vi "State Convert for Save.vi"(6 "Control Ref Queue":T1, 8 "error in (no error)":errorcluster, 11 "2D Plot.lvclass":refnum<class "2D Plot.lvclass">) -> (0 "error out":errorcluster, 1 "Plot Legend Color":u32(colorbox), 2 "Main Frame Color":u32(colorbox), 3 "2D Plot.lvclass out":refnum<class "2D Plot.lvclass">)   [LabVIEW 2017, in "2D Plot.lvclass"]
uses:
  <vilib>/Math Plots/2D Math Plots/2D Plot/2D Plot/2D Plot.lvclass
  <vilib>/Math Plots/2D Math Plots/2D Plot/Action String/2DMathPlot Ctrl Act Queue.ctl
  <vilib>/Math Plots/2D Math Plots/2D Plot/Action String/2DMathPlot Ctrl Act Cluster.ctl
  <vilib>/Math Plots/2D Math Plots/2D Plot/Action String/2DMathPlot State Class.ctl
  <vilib>/Math Plots/2D Math Plots/2D Plot/2D Plot/2D Plot.lvclass/2D Plot.ctl
  <vilib>/Math Plots/Plot Private Lib/NI_Math Plot Private Lib.lvlib
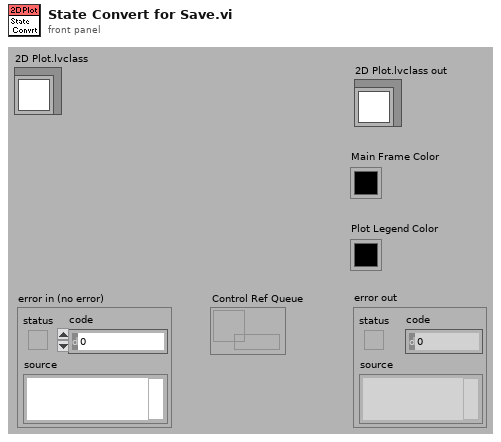
[diagram p1: front panel]
types:
  T1 = typedef "2DMathPlot Ctrl Act Queue.ctl" = refnum<queue>
  T2 = typedef "2DMathPlot Ctrl Act Cluster.ctl" = cluster{"Plot Area Ref":refnum<vi>, "Z Axis Ref":refnum<vi>, "Legend Ref":refnum<vi>, "XControl Ref":refnum<vi>, "Facade Ref":refnum<vi>, "Display State Change Class":T3}
  T3 = typedef "2DMathPlot State Class.ctl" = enum16{"Update All (Undo)", "Update General", "Update Appearance", "Update Format", "Update Scale", "Update Marker", "Update Cursor", "None"}
  T4 = typedef "LVRectTypeDef.ctl" = cluster{"Left":i16, "Top":i16, "Right":i16, "Bottom":i16}
  T5 = typedef "LVAnnotationListTypeDef.ctl" = cluster{"Name":string, "Color":u32, "Style":u8, "Point Style":u8, "Name Visible":bool, "Allow Drag":bool, "Annotation Mode":u32, "Plot":i32, "Index":i32, "Position":cluster{"X":dbl, "Y":dbl}, "X Scale":u32, "Y Scale":u32, "Show Arrow":bool, "Lock Name":bool, "Plot Area":i32, "Label Offset":cluster{"X":dbl, "Y":dbl}}[]
  T6 = typedef "LVCursorListTypeDef.ctl" = cluster{"Name":string, "Color":u32, "Style":u8, "Point Style":u8, "Name Visible":bool, "Allow Drag":bool, "Cursor Mode":u32, "Plot":i32, "Index":i32, "Position":cluster{"X":dbl, "Y":dbl}, "X Scale":u32, "Y Scale":u32, "Watch Plots":i32[], "Watch All Plots":bool, "Plot Area":i32, "Label Offset":cluster{"X":dbl, "Y":dbl}}[]
  T7 = cluster{"Cursor Selection Color":u32, "Line Style":u8, "Line Width":u8, "Visible":bool}
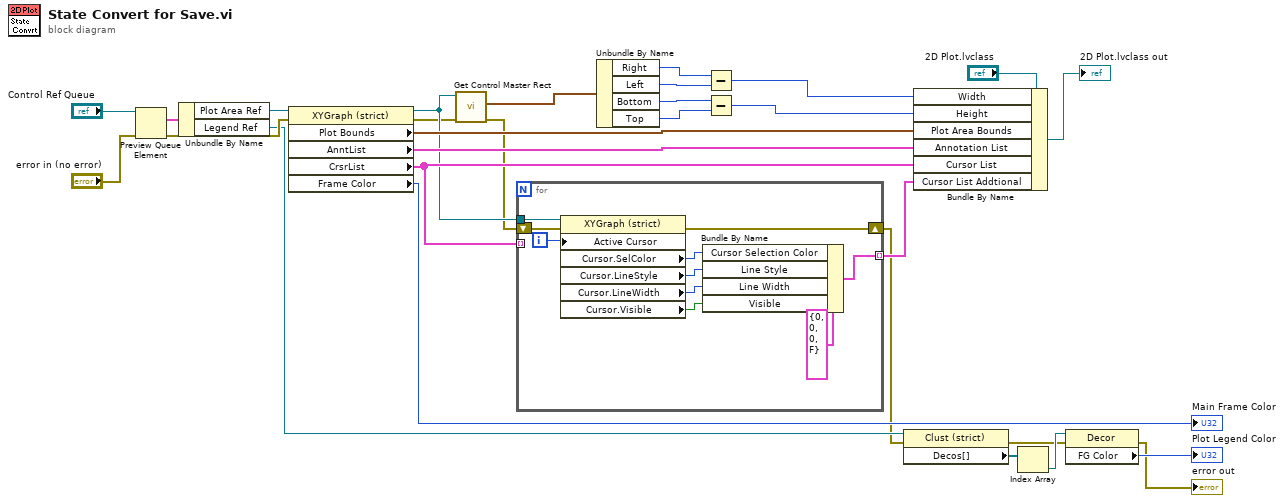
[diagram p0: block diagram]
diagram:
  n1 = Preview Queue Element(queue="Control Ref Queue", error in (no error)="error in (no error)") -> (element=w25:T2, error out=w27:errorcluster)  [unwired: 3 out]
  n2 = Unbundle By Name(w25) -> ("Plot Area Ref"=w26:refnum<vi>, "Legend Ref"=w3:refnum<vi>)
  n3 = property class="XYGraph (strict)"(reference=w26, error in=w27) -> (reference out=w11:refnum<vi>, error out=w10:errorcluster, "Plot Bounds"=w20:T4, "AnntList"=w19:T5, "CrsrList"=w29:T6, "Frame Color"=→"Main Frame Color":u32)
  n4 = call <vilib>:"Get Control Master Rect.vi"("error in (no error)"=w10, "reference"=w11) -> ("error out"=w9:errorcluster, "Master Bounds Rect"=w12:T4)  [unwired: 8 out]
  n5 = for {
    tunnel: w11 -> [w39]
    shift-right: [w36] -> w2
    shift-left: w9 -> [w37]
    tunnel: [w30] -> w28 mode=indexing
    tunnel: w29 -> [_] mode=indexing
    i -> [w38]
    n6 = property class="XYGraph (strict)"(reference=w39, error in=w37, "Active Cursor"=w38) -> (error out=w36:errorcluster, "Cursor.SelColor"=w34:u32, "Cursor.LineStyle"=w33:u8, "Cursor.LineWidth"=w32:u8, "Cursor.Visible"=w31:bool)  [unwired: 1 out]
    n7 = Bundle By Name(cluster=T7 {"Cursor Selection Color"=0, "Line Style"=0, "Line Width"=0, "Visible"=FALSE} ("Rest Attribute"), "Cursor Selection Color"=w34, "Line Style"=w33, "Line Width"=w32, "Visible"=w31) -> (w30:T7)
  }
  n8 = Unbundle By Name(w12) -> ("Right"=w15:i16, "Left"=w16:i16, "Bottom"=w17:i16, "Top"=w18:i16)
  n9 = Subtract(x=w15, y=w16) -> (x-y=w14:i16)
  n10 = Subtract(x=w17, y=w18) -> (x-y=w13:i16)
  n11 = property class="Clust (strict)"(reference=w3, error in=w2) -> (error out=w6:errorcluster, "Decos[]"=w7:refnum<vi>[])  [unwired: 1 out]
  n12 = Bundle By Name(cluster="2D Plot.lvclass", "Width"=w14, "Height"=w13, "Plot Area Bounds"=w20, "Annotation List"=w19, "Cursor List"=w29, "Cursor List Addtional"=w28) -> (→"2D Plot.lvclass out":refnum<class "2D Plot.lvclass">)
  n13 = Index Array(array=w7) -> (element=w8:refnum<vi>)  [unwired: 1 in]
  n14 = property class="Decor"(reference=w8, error in=w6) -> (error out=→"error out":errorcluster, "FG Color"=→"Plot Legend Color":u32)  [unwired: 1 out]
